vi "MGI Filter Error[].vi"(9 "Ignore Warnings? (F: Process Errors and Warnings)":bool, 10 "Error Occurence[]":errorcluster[](array[cluster]), 11 "MGI Error Reporter Base in":refnum<class "MGI Error Reporter Base.lvclass">) -> (2 "Filtered Error[]":errorcluster[](array[cluster]), 3 "MGI Error Reporter Base out":refnum<class "MGI Error Reporter Base.lvclass">)   [LabVIEW 2016, in "MGI Error Reporter Base.lvclass"]
doc: "Filter the input Error[]. Child class may override this VI, which filters Warnings if \"Ignore Warnings?\" is true.\n\nAuthored by Shawn Walpole\nsupport@mooregoodideas.com\nwww.mooregoodideas.com\n\nCopyright (c) 2013, Moore Good Ideas, Inc.\n\nAll rights reserved.\n\nRedistribution and use in source and binary forms, with or without modification, are permitted provided that the following conditions are met:\n\n * Redistributions of source code must retain the above copyright notice, this list of conditions and the following disclaimer.\n * Redistributions in binary form must reproduce the above copyright notice, this list of conditions and the following disclaimer in the documentation and/or other materials provided with the distribution.\n * Neither the name of Moore Good Ideas, Inc. nor the names of its contributors may be used to endorse or promote products derived from this software without specific prior written permission.\n\nTHIS SOFTWARE IS PROVIDED BY THE COPYRIGHT HOLDERS AND CONTRIBUTORS \"AS IS\" AND ANY EXPRESS OR IMPLIED WARRANTIES, INCLUDING, BUT NOT LIMITED TO, THE IMPLIED WARRANTIES OF MERCHANTABILITY AND FITNESS FOR A PARTICULAR PURPOSE ARE DISCLAIMED. IN NO EVENT SHALL THE COPYRIGHT OWNER OR CONTRIBUTORS BE LIABLE FOR ANY DIRECT, INDIRECT, INCIDENTAL, SPECIAL, EXEMPLARY, OR CONSEQUENTIAL DAMAGES (INCLUDING, BUT NOT LIMITED TO, PROCUREMENT OF SUBSTITUTE GOODS OR SERVICES; LOSS OF USE, DATA, OR PROFITS; OR BUSINESS INTERRUPTION) HOWEVER CAUSED AND ON ANY THEORY OF LIABILITY, WHETHER IN CONTRACT, STRICT LIABILITY, OR TORT (INCLUDING NEGLIGENCE OR OTHERWISE) ARISING IN ANY WAY OUT OF THE USE OF THIS SOFTWARE, EVEN IF ADVISED OF THE POSSIBILITY OF SUCH DAMAGE."
uses:
  <userlib>/_MGI/Error Reporter/MGI Error Reporter Base/MGI Error Reporter Base.lvclass
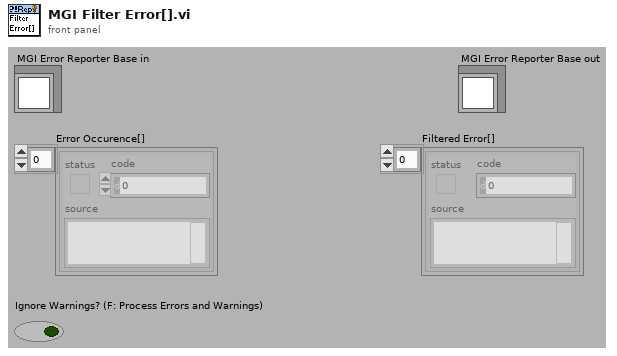
[diagram p1: front panel]
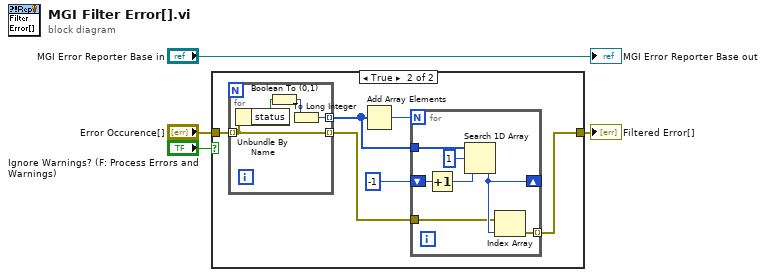
[diagram p0: block diagram]
diagram:
  n1 = case shown="True" "Ignore Warnings? (F: Process Errors and Warnings)" {
    tunnel: "Error Occurence[]" -> [w5 w11]
    tunnel: [w5 w6] -> w1
    frame False {
    }
    frame True {
      n2 = for {
        tunnel: w11 -> [w22] mode=indexing
        tunnel: [w22] -> w8 mode=indexing
        tunnel: [w19] -> w7 mode=indexing
        n3 = Unbundle By Name(w22) -> ("status"=w21:bool)
        n4 = Boolean To (0,1)(Boolean=w21) -> (0, 1=w20:i16)
        n5 = To Long Integer(number=w20) -> (32bit integer=w19:i32)
      }
      n6 = Add Array Elements(numeric array=w7) -> (sum=w9:i32)
      n7 = for {
        N: w9 -> [_]
        tunnel: w8 -> [w15]
        tunnel: w7 -> [w18]
        shift-right: [w16] -> _
        shift-left: -1 ("start index (0)") -> [w17]
        tunnel: [w14] -> w6 mode=indexing
        n8 = Increment(x=w17) -> (x+1=w13:i32)
        n9 = Search 1D Array(1D array=w18, element=1, start index (0)=w13) -> (index of element=w16:i32)
        n10 = Index Array(array=w15, index=w16) -> (element=w14:errorcluster)
      }
    }
  }
  "Filtered Error[]" <- w1
  "MGI Error Reporter Base out" <- "MGI Error Reporter Base in"
